vi "Array_Avg_5pt.vi"(1 "array":dbl[](array[numeric])) -> (0 "Value out":dbl)   [LabVIEW 2014]
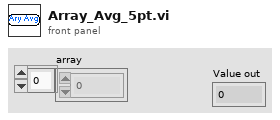
[diagram p1: front panel]
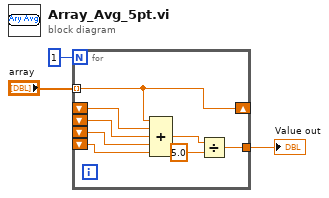
[diagram p0: block diagram]
diagram:
  n1 = for {
    N: 1 -> [_]
    tunnel: "array" -> [w11] mode=indexing
    shift-right: [w11] -> _
    shift-left: _ -> [w10]
    shift-left: _ -> [w9]
    tunnel: [w6] -> w2
    shift-left: _ -> [w5]
    shift-left: _ -> [w4]
    n2 = Compound Arithmetic op=ADD(w11, w10, w9, w5, w4) -> (w8:dbl)
    n3 = Divide(x=w8, y=5.0) -> (x/y=w6:dbl)
  }
  "Value out" <- w2
